vi "WriteIniFile.vi"(1 "Section":string="AzCamTool", 2 "value":string, 3 "key":string) -> (0 "Error":errorcluster)   [LabVIEW 2014]
uses:
  globals/AzCamGlobals.vi
  <vilib>/Utility/config.llb/Write Key (String).vi
  <vilib>/Utility/config.llb/NI_LVConfig.lvlib
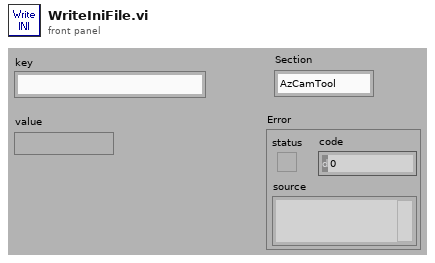
[diagram p1: front panel]
types:
  T1 = typedef "NI_LVConfig.lvlib/Config Data RefNum.ctl" = refnum<k1>
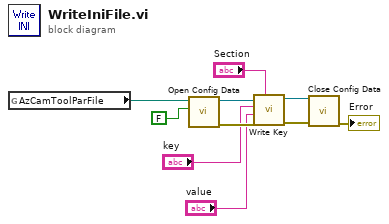
[diagram p0: block diagram]
diagram:
  n1 = global read "AzCamGlobals.vi" "AzCamToolParFile"() -> (w2:path)
  n2 = call <vilib>:"Open Config Data.vi"("create file if necessary (T)"=FALSE ("create file if necessary? (T)"), "configuration file path"=w2) -> ("error out"=w7:errorcluster, "refnum"=w10:T1)  [unwired: 7 in, 1 out]
  n3 = call-poly <vilib>:"Write Key.vi"("section"="Section", "error in (no error)"=w7, "value"="value", "key"="key", "refnum"=w10) -> ("error out"=w5:errorcluster, "refnum out"=w6:T1)  [unwired: 4 in, 1 out]
  n4 = call <vilib>:"Close Config Data.vi"("error in (no error)"=w5, "refnum"=w6) -> ("error out"=→"Error":errorcluster)  [unwired: 8 in, 1 out]
